vi "Controller Write PS Filter Enable.vi"(0 "PS Filter Enable":refnum<k21>[](array[refnum]), 5 "Filter Enable":bool, 11 "error in":errorcluster) -> (15 "error out":errorcluster)   [LabVIEW 2011]
uses:
  Controller VIs.lvlib
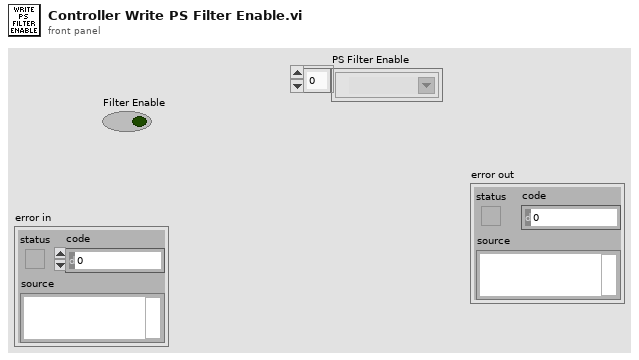
[diagram p1: front panel]
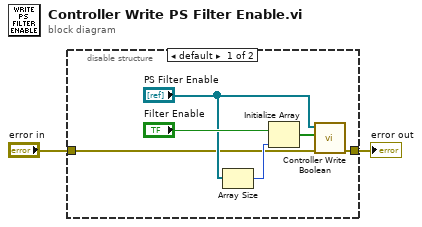
[diagram p0: block diagram]
diagram:
  n1 = disable-structure shown="default" {
    disable-tunnel: "error in" -> [w4 _]
    disable-tunnel: [w3 _] -> w1
    frame condition #0 (active) {
      n2 = Array Size(array="PS Filter Enable") -> (size(s)=w6:i32)
      n3 = Initialize Array("Filter Enable", w6) -> (w7:bool[])
      n4 = call "Controller Write Boolean.vi"("Error In"=w4, "Values"=w7, "Variables"="PS Filter Enable") -> ("Error Out"=w3:errorcluster)  [unwired: 8 in]
    }
    frame condition #1 {
    }
  }
  "error out" <- w1
